vi "KeyReader.vi"() -> ()   [LabVIEW 2019]
uses:
  <vilib>/Utility/inputDevices.llb/keyboardAcquire.vi
panel:
  in  "stop":bool
  out "error out":errorcluster
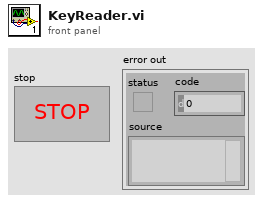
[diagram p1: front panel]
types:
  T1 = enum16{"0", "1", "2", "3", "4", "5", "6", "7", "8", "9", "A", "B", "C", "D", "E", "F", "G", "H", "I", "J", "K", "L", "M", "N", "O", "P", "Q", "R", "S", "T", "U", "V", "W", "X", "Y", "Z", "F1", "F2", "F3", "F4", "F5", "F6", "F7", "F8", "F9", "F10", "F11", "F12", "F13", "F14", "F15", "ADD", "BACK", "BACKSLASH", "CAPITAL", "COMMA", "DECIMAL", "DELETE", "DIVIDE", "DOWN", "END", "EQUALS", "ESCAPE", "GRAVE (`)", "HOME", "INSERT", "LBRACKET", "LCONTROL", "LEFT", "L ALT", "LSHIFT", "LWIN", "MINUS", "MULTIPLY", "NEXT", "NUMLOCK", "NUMPAD_0", "NUMPAD_1", "NUMPAD_2", "NUMPAD_3", "NUMPAD_4", "NUMPAD_5", "NUMPAD_6", "NUMPAD_7", "NUMPAD_8", "NUMPAD_9", "PAUSE", "PERIOD", "PRIOR (PG UP)", "RBRACKET", "RCONTROL", "RETURN", "RIGHT", "R ALT", "RSHIFT", "RWIN", "SCROLL", "SEMICOLON", "SLASH", "SPACE", "SUBTRACT", "TAB", "UP", "ENTER (num pad)", "' (quote)"}[]
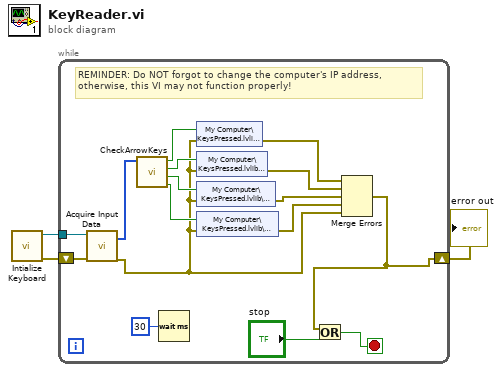
[diagram p0: block diagram]
diagram:
  n1 = call <vilib>:"Intialize Keyboard.vi"() -> ("error out"=w3:errorcluster, "device ID"=w2:refnum<k1>)  [unwired: 10 in]
  n2 = while {
    tunnel: w2 -> [w18]
    shift-right: [w5] -> w1
    shift-left: w3 -> [w19]
    stop <- w16 stop-if-true
    # "REMINDER: Do NOT forgot to change the computer's IP address,\notherwise, this VI may not function properly!"
    n3 = call-poly <vilib>:"Acquire Input Data.vi"("device ID"=w18, "error in (no error)"=w19) -> ("keys pressed"=w17:T1, "error out"=w10:errorcluster)  [unwired: 15 in, 1 out]
    n4 = call "CheckArrowKeys.vi"("Array"=w17) -> ("Down"=w11:bool, "Right"=w12:bool, "Left"=w13:bool, "Up"=w14:bool)  [unwired: 6 in, 1 out]
    n5 = Wait (ms)(milliseconds to wait=u32 30) -> ()  [unwired: 1 out]
    n6 = shared-variable "My Computer\\KeysPressed.lvlib\\Up1"(w14, error in=w10) -> (error out=w6:errorcluster)
    n7 = shared-variable "My Computer\\KeysPressed.lvlib\\Left1"(w13, error in=w10) -> (error out=w7:errorcluster)
    n8 = shared-variable "My Computer\\KeysPressed.lvlib\\Right1"(w12, error in=w10) -> (error out=w8:errorcluster)
    n9 = shared-variable "My Computer\\KeysPressed.lvlib\\Down1"(w11, error in=w10) -> (error out=w9:errorcluster)
    n10 = Merge Errors(w6, w7, w8, w9, w10) -> (w5:errorcluster)
    n11 = Or(x=w5, y="stop") -> (x .or. y?=w16:bool)
  }
  "error out" <- w1
